vi "Execute.vi"(8 "error in (no error)":errorcluster, 9 "Sequence Parameters in":variant, 11 "Example Step One in":refnum<class "Example Step One.lvclass">) -> (0 "error out":errorcluster, 1 "Sequence Parameters out":variant, 3 "Example Step One out":refnum<class "Example Step One.lvclass">)   [LabVIEW 2015, in "Mediator.lvlib" / "Example Step One.lvclass"]
doc: "This determines what action is performed when this step is run.s"
uses:
  Example Step One.lvclass
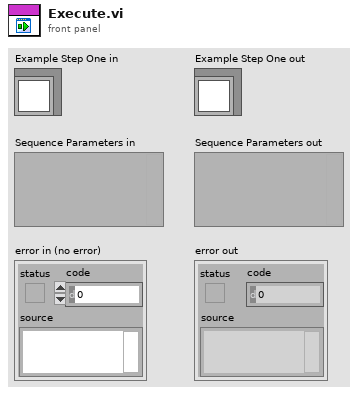
[diagram p1: front panel]
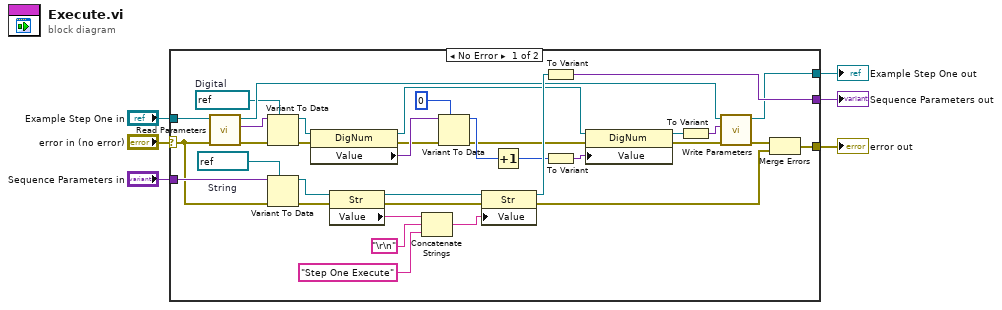
[diagram p0: block diagram]
diagram:
  n1 = case shown="No Error" "error in (no error)" {
    selector: "error in (no error)" -> [w21 w43]
    tunnel: [w22 w43] -> w5
    tunnel: "Sequence Parameters in" -> [w41 w42]
    tunnel: "Example Step One in" -> [w29 w44]
    tunnel: [w27 w44] -> w2
    tunnel: [w33 w42] -> w1
    frame No Error {
      w19 = refnum<vi> refnum  # Digital
      w40 = refnum<vi> refnum  # String
      n2 = call-dynamic "Read Parameters.vi"("error in (no error)"=w21, "Step in"=w29) -> ("error out"=w20:errorcluster, "Parameters"=w26:variant, "Step out"=w28:refnum<class "Example Step One.lvclass">)  [unwired: 7 in]
      n3 = Variant To Data(error in=w20, type=w19, Variant=w26) -> (data=w18:refnum<vi>, error out=w10:errorcluster)
      n4 = Variant To Data(error in=w21, type=w40, Variant=w41) -> (data=w39:refnum<vi>, error out=w31:errorcluster)
      n5 = property class="DigNum"(reference=w18, error in=w10) -> (reference out=w12:refnum<vi>, error out=w9:errorcluster, "Value"=w17:variant)
      n6 = property class="Str"(reference=w39, error in=w31) -> (reference out=w35:refnum<vi>, error out=w30:errorcluster, "Value"=w38:string)
      n7 = Concatenate Strings(w38, "\r\n", "Step One Execute" ("string")) -> (w34:string)
      n8 = Variant To Data(error in=w9, type=0, Variant=w17) -> (data=w15:i32, error out=w8:errorcluster)
      n9 = property class="Str"(reference=w35, error in=w30, "Value"=w34) -> (reference out=w32:refnum<vi>, error out=w23:errorcluster)
      n10 = Increment(x=w15) -> (x+1=w14:i32)
      n11 = To Variant(anything=w32) -> (Variant=w33:variant)
      n12 = To Variant(anything=w14) -> (Variant=w13:variant)
      n13 = property class="DigNum"(reference=w12, error in=w8, "Value"=w13) -> (reference out=w11:refnum<vi>, error out=w7:errorcluster)
      n14 = To Variant(anything=w11) -> (Variant=w25:variant)
      n15 = call-dynamic "Write Parameters.vi"("error in (no error)"=w7, "Parameters"=w25, "Step in"=w28) -> ("error out"=w24:errorcluster, "Step out"=w27:refnum<class "Example Step One.lvclass">)  [unwired: 7 in]
      n16 = Merge Errors(w24, w23) -> (w22:errorcluster)
    }
    frame Error {
    }
  }
  "error out" <- w5
  "Example Step One out" <- w2
  "Sequence Parameters out" <- w1
